vi "Get diagnostics lists.vi"(8 "error in (no error)":errorcluster, 11 "UIParameters.DiagnosticsParameters":T2) -> (0 "error out":errorcluster, 3 "Diagnostics details":T1)   [LabVIEW 2019, in "ZenGage v3.0 UI.lvclass"]
uses:
  ZenGage v3.0 UI.lvclass
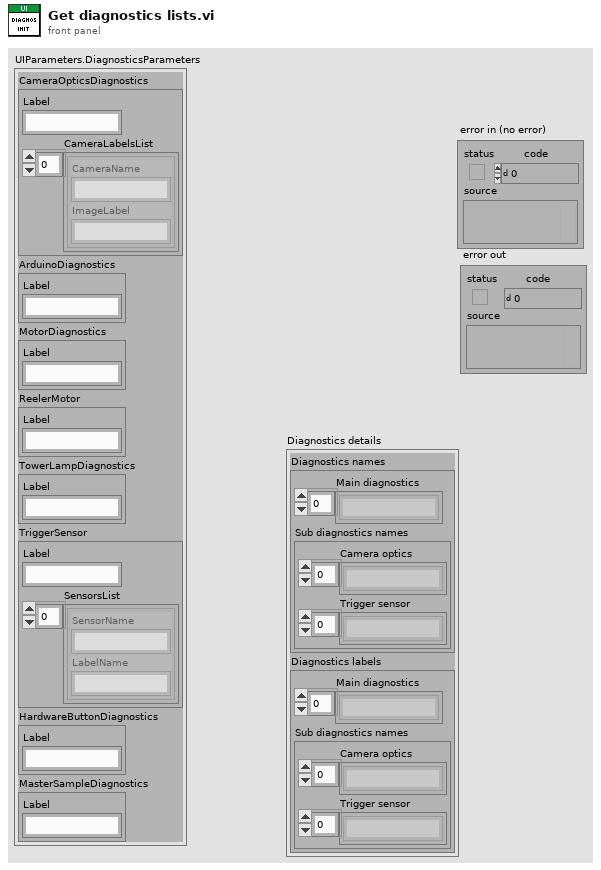
[diagram p1: front panel]
types:
  T1 = cluster{"Diagnostics names":cluster{"Main diagnostics":string[], "Sub diagnostics names":cluster{"Camera optics":string[], "Trigger sensor":string[]}}, "Diagnostics labels":cluster{"Main diagnostics":string[], "Sub diagnostics names":cluster{"Camera optics":string[], "Trigger sensor":string[]}}}
  T2 = cluster{"CameraOpticsDiagnostics":cluster{"Label":string, "CameraLabelsList":cluster{"CameraName":string, "ImageLabel":string}[]}, "ArduinoDiagnostics":cluster{"Label":string}, "MotorDiagnostics":cluster{"Label":string}, "ReelerMotor":cluster{"Label":string}, "TowerLampDiagnostics":cluster{"Label":string}, "TriggerSensor":cluster{"Label":string, "SensorsList":cluster{"SensorName":string, "LabelName":string}[]}, "HardwareButtonDiagnostics":cluster{"Label":string}, "MasterSampleDiagnostics":cluster{"Label":string}}
  T3 = cluster{"Label":string, "CameraLabelsList":cluster{"CameraName":string, "ImageLabel":string}[]}
  T4 = cluster{"Label":string, "SensorsList":cluster{"SensorName":string, "LabelName":string}[]}
  T5 = cluster{"CameraName":string, "ImageLabel":string}[]
  T6 = cluster{"SensorName":string, "LabelName":string}[]
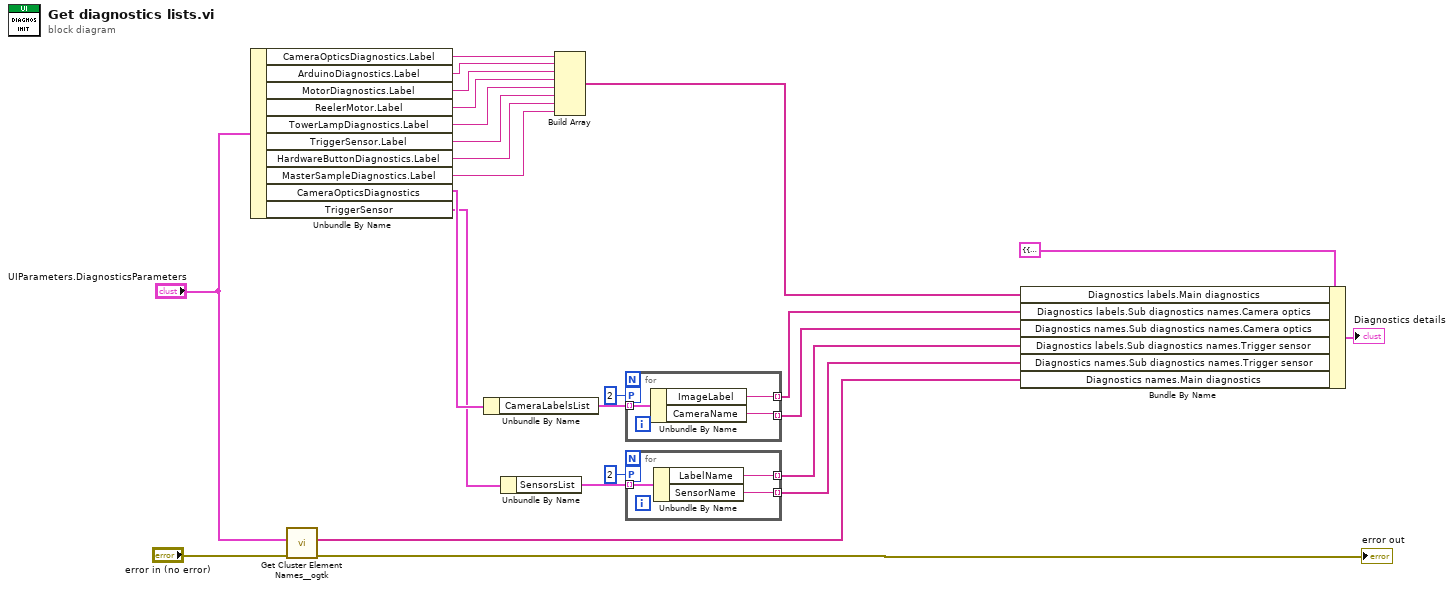
[diagram p0: block diagram]
diagram:
  n1 = Unbundle By Name("UIParameters.DiagnosticsParameters") -> ("CameraOpticsDiagnostics.Label"=w9:string, "ArduinoDiagnostics.Label"=w8:string, "MotorDiagnostics.Label"=w7:string, "ReelerMotor.Label"=w6:string, "TowerLampDiagnostics.Label"=w5:string, "TriggerSensor.Label"=w4:string, "HardwareButtonDiagnostics.Label"=w3:string, "MasterSampleDiagnostics.Label"=w2:string, "CameraOpticsDiagnostics"=w25:T3, "TriggerSensor"=w24:T4)
  n2 = call <userlib>:"Get Cluster Element Names__ogtk.vi"("error in (no error)"="error in (no error)", "Cluster"="UIParameters.DiagnosticsParameters") -> ("error out"=→"error out":errorcluster, "Element Names"=w12:string[])  [unwired: 8 in]
  n3 = Unbundle By Name(w25) -> ("CameraLabelsList"=w23:T5)
  n4 = Unbundle By Name(w24) -> ("SensorsList"=w22:T6)
  n5 = Build Array(w9, w8, w7, w6, w5, w4, w3, w2) -> (w1:string[])
  n6 = for {
    tunnel: w23 -> [w28] mode=indexing
    tunnel: [w27] -> w16 mode=indexing
    tunnel: [w26] -> w15 mode=indexing
    workers-P: 2 -> [_]
    n7 = Unbundle By Name(w28) -> ("ImageLabel"=w27:string, "CameraName"=w26:string)
  }
  n8 = for {
    tunnel: w22 -> [w31] mode=indexing
    tunnel: [w30] -> w14 mode=indexing
    tunnel: [w29] -> w13 mode=indexing
    workers-P: 2 -> [_]
    n9 = Unbundle By Name(w31) -> ("LabelName"=w30:string, "SensorName"=w29:string)
  }
  n10 = Bundle By Name(cluster=T1 {"Diagnostics names"={"Main diagnostics"=[], "Sub diagnostics names"={"Camera optics"=[], "Trigger sensor"=[]}}, "Diagnostics labels"={"Main diagnostics"=[], "Sub diagnostics names"={"Camera optics"=[], "Trigger sensor"=[]}}} ("Diagnostics.Diagnostics details"), "Diagnostics labels.Main diagnostics"=w1, "Diagnostics labels.Sub diagnostics names.Camera optics"=w16, "Diagnostics names.Sub diagnostics names.Camera optics"=w15, "Diagnostics labels.Sub diagnostics names.Trigger sensor"=w14, "Diagnostics names.Sub diagnostics names.Trigger sensor"=w13, "Diagnostics names.Main diagnostics"=w12) -> (→"Diagnostics details":T1)
